vi "RemoveMission.vi"(8 "error in (no error)":errorcluster, 9 "NotifierReff":T1, 10 "ID to delete":i32, 11 "Mission Notifier":refnum<notifier>) -> (0 "error out":errorcluster)   [LabVIEW 2013]
doc: "This VI removes an Mission with an indicated ID from the notifier array that it was stored in.\n\nEric Schneider, August 2014"
uses:
  Classes/Missions/GenericMission/GenericMission.lvclass
  Data/TypeDefs/Notifiers.ctl
  Data/TypeDefs/UTM Location.ctl
  Data/TypeDefs/Sail Set Suggestions.ctl
  Data/TypeDefs/Rudder Set Suggestions.ctl
  Data/TypeDefs/OverrideInformation.ctl
  Data/TypeDefs/OverrideMode.ctl
  Data/TypeDefs/MotorSetup.ctl
  Data/TypeDefs/DynamixelSetupInfo.ctl
  Data/TypeDefs/AirmarStatus.ctl
  Data/TypeDefs/HardwareOnline.ctl
  Data/TypeDefs/DynamixelCycleTracker.ctl
  Data/TypeDefs/RC Input Values.ctl
  Classes/Waypoint/Waypoint.lvclass
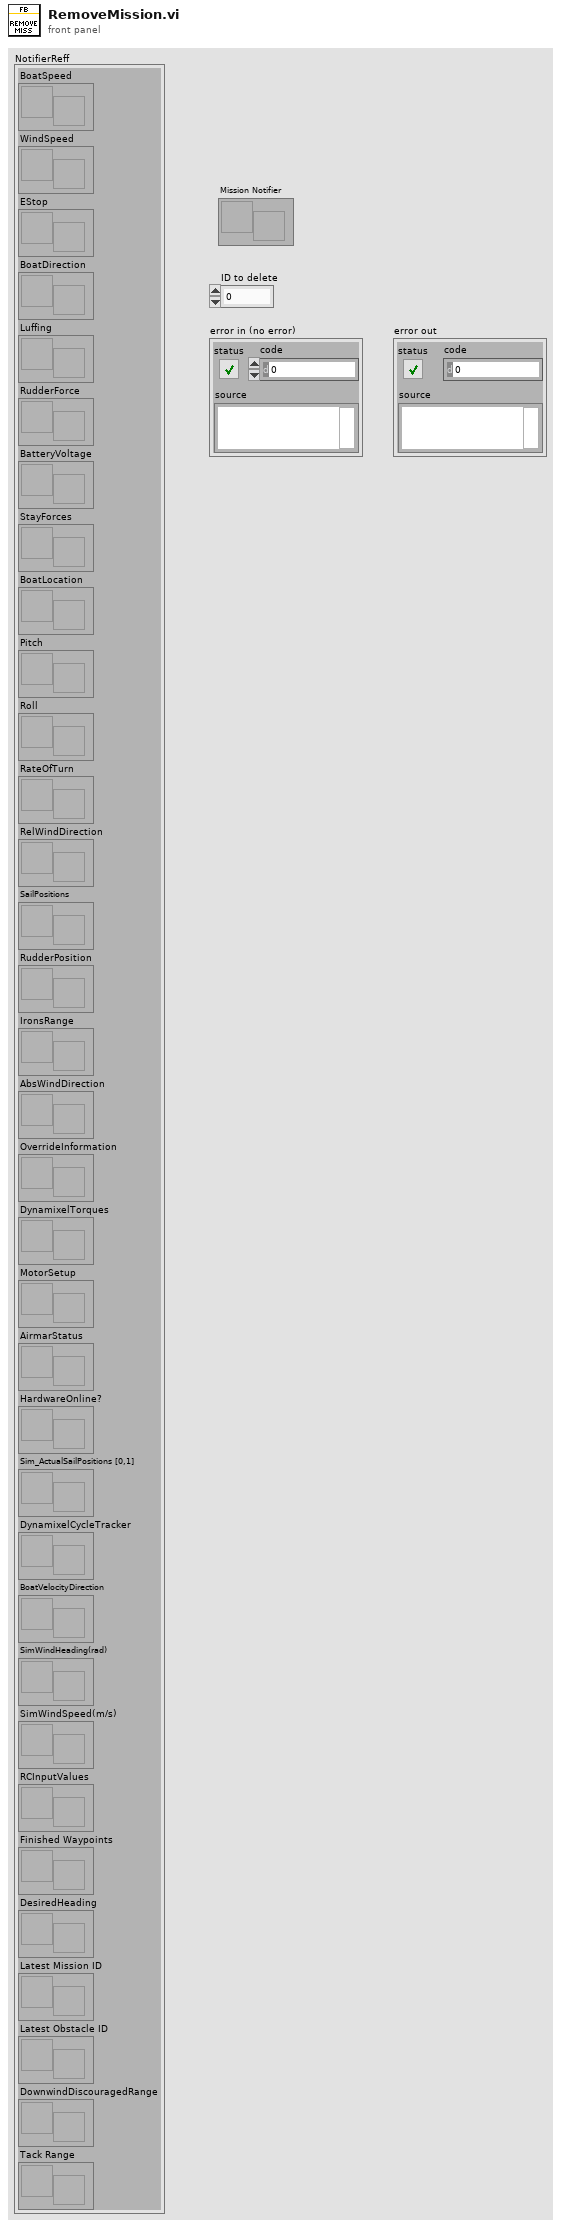
[diagram p1: front panel]
types:
  T1 = typedef "Notifiers.ctl" = cluster{"BoatSpeed":refnum<notifier>, "WindSpeed":refnum<notifier>, "EStop":refnum<notifier>, "BoatDirection":refnum<notifier>, "Luffing":refnum<notifier>, "RudderForce":refnum<notifier>, "BatteryVoltage":refnum<notifier>, "StayForces":refnum<notifier>, "BoatLocation":refnum<notifier>, "Pitch":refnum<notifier>, "Roll":refnum<notifier>, "RateOfTurn":refnum<notifier>, "RelWindDirection":refnum<notifier>, "SailPositions":refnum<notifier>, "RudderPosition":refnum<notifier>, "IronsRange":refnum<notifier>, "AbsWindDirection":refnum<notifier>, "OverrideInformation":refnum<notifier>, "DynamixelTorques":refnum<notifier>, "MotorSetup":refnum<notifier>, "AirmarStatus":refnum<notifier>, "HardwareOnline?":refnum<notifier>, "Sim_ActualSailPositions [0,1]":refnum<notifier>, "DynamixelCycleTracker":refnum<notifier>, "BoatVelocityDirection":refnum<notifier>, "SimWindHeading(rad)":refnum<notifier>, "SimWindSpeed(m/s)":refnum<notifier>, "RCInputValues":refnum<notifier>, "Finished Waypoints":refnum<notifier>, "DesiredHeading":refnum<notifier>, "Latest Mission ID":refnum<notifier>, "Latest Obstacle ID":refnum<notifier>, "DownwindDiscouragedRange":refnum<notifier>, "Tack Range":refnum<notifier>}
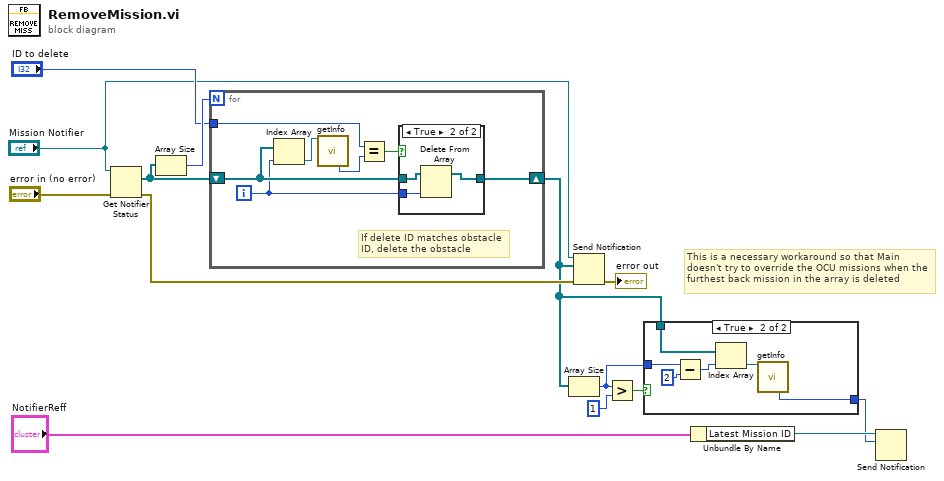
[diagram p0: block diagram]
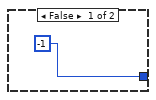
[diagram p2: hidden frame]
diagram:
  # "This is a necessary workaround so that Main doesn't try to override the OCU missions when the furthest back mission in the array is deleted"
  n1 = Get Notifier Status(notifier="Mission Notifier", error in (no error)="error in (no error)") -> (current notification=w12:refnum<class "GenericMission.lvclass">[], error out=w14:errorcluster)  [unwired: 3 out]
  n2 = Array Size(array=w12) -> (size(s)=w11:i32)
  n3 = for {
    N: w11 -> [_]
    tunnel: "ID to delete" -> [w19]
    shift-right: [w17] -> w4
    shift-left: w12 -> [w21]
    i -> [w18]
    # "If delete ID matches obstacle ID, delete the obstacle"
    n4 = Index Array(array=w21, index=w18) -> (element=w16:refnum<class "GenericMission.lvclass">)
    n5 = call-dynamic "getInfo.vi"("GenericMission in"=w16) -> ("ID#"=w15:i16)  [unwired: 6 in, 8 out]
    n6 = Equal?(x=w19, y=w15) -> (x = y?=w20:bool)
    n7 = case shown="True" w20 {
      tunnel: w21 -> [w22 w25]
      tunnel: w18 -> [_ w24]
      tunnel: [w22 w23] -> w17
      frame False {
      }
      frame True {
        n8 = Delete From Array(array=w25, index=w24) -> (array with subset deleted=w23:refnum<class "GenericMission.lvclass">[])  [unwired: 1 in, 1 out]
      }
    }
  }
  n9 = Array Size(array=w4) -> (size(s)=w3:i32)
  n10 = Send Notification(notification=w4, notifier="Mission Notifier", error in (no error)=w14) -> (error out=→"error out":errorcluster)  [unwired: 1 out]
  n11 = Greater?(x=w3, y=1) -> (0:w5:bool)
  n12 = case shown="True" w5 {
    tunnel: w4 -> [_ w32]
    tunnel: w3 -> [_ w31]
    tunnel: [i16 -1 ("ID#") w27] -> w1
    frame False {
    }
    frame True {
      n13 = Subtract(x=w31, y=2) -> (x-y=w29:i32)
      n14 = Index Array(array=w32, index=w29) -> (element=w28:refnum<class "GenericMission.lvclass">)
      n15 = call-dynamic "getInfo.vi"("GenericMission in"=w28) -> ("ID#"=w27:i16)  [unwired: 6 in, 8 out]
    }
  }
  n16 = Unbundle By Name("NotifierReff") -> ("Latest Mission ID"=w2:refnum<notifier>)
  n17 = Send Notification(notification=w1, notifier=w2) -> ()  [unwired: 1 in, 2 out]
